vi "Translator.Translate.Text.New.vi"(6 "group":string, 8 "error in (no error)":errorcluster, 10 "text":string) -> (0 "error out":errorcluster, 2 "translated":string)   [LabVIEW 2019, in "Tools.lvlib"]
uses:
  Tools.lvlib
  TMOS config/TMOS.Config.Action.ctl
  <vilib>/Utility/config.llb/NI_LVConfig.lvlib
  Translator.File.MatchStrings (Single).vi
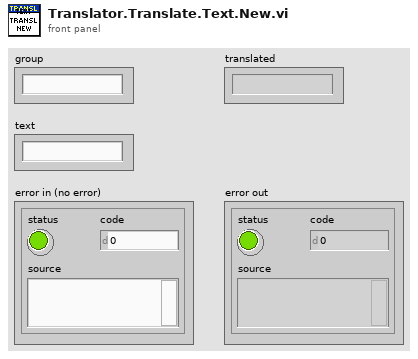
[diagram p1: front panel]
types:
  T1 = typedef "TMOS.Config.Action.ctl" = enum16{"init", "update", "get", "set"}
  T2 = typedef "NI_LVConfig.lvlib/Config Data RefNum.ctl" = refnum<k1>
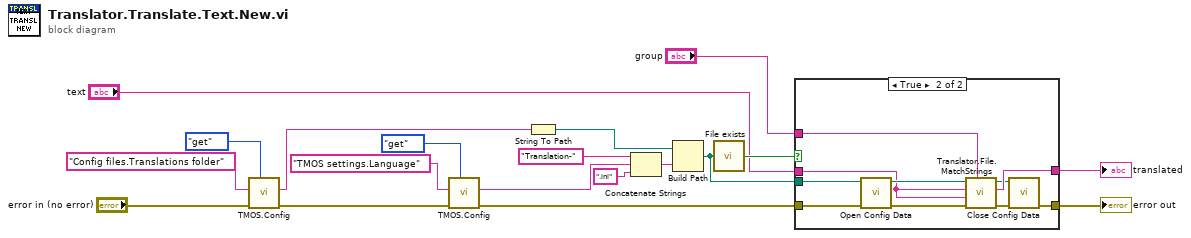
[diagram p0: block diagram]
diagram:
  n1 = call "TMOS.Config.vi"("action"=TMOS.Config.Action."get", "error in"="error in (no error)", "name"="Config files.Translations folder" ("~Language in use")) -> ("error out"=w16:errorcluster, "read value"=w13:string)  [unwired: 6 in, 1 out]
  n2 = call "TMOS.Config.vi"("action"=TMOS.Config.Action."get", "error in"=w16, "name"="TMOS settings.Language" ("~Language in use")) -> ("error out"=w4:errorcluster, "read value"=w9:string)  [unwired: 6 in, 1 out]
  n3 = String To Path(string=w13) -> (path=w8:path)
  n4 = Concatenate Strings("Translation-" ("string"), w9, ".ini" ("string")) -> (w12:string)
  n5 = Build Path(base path=w8, name or relative path=w12) -> (appended path=w5:path)
  n6 = call "File exists.vi"("file path"=w5) -> ("exists?"=w6:bool)  [unwired: 4 in]
  n7 = case shown="True" w6 {
    tunnel: w5 -> [_ w22]
    tunnel: w4 -> [w21 w31]
    tunnel: "text" -> [w20 w28]
    tunnel: [w20 w27] -> w1
    tunnel: [w21 w24] -> w2
    tunnel: "group" -> [_ w23]
    frame False {
    }
    frame True {
      n8 = call <vilib>:"Open Config Data.vi"("error in (no error)"=w31, "configuration file path"=w22) -> ("error out"=w29:errorcluster, "refnum"=w30:T2)  [unwired: 7 in, 1 out]
      n9 = call-poly "Translator.File.MatchStrings.vi"("group"=w23, "error in"=w29, "label"=w28, "default value"=w28, "refnum in"=w30) -> ("error out"=w26:errorcluster, "value out"=w27:string, "refnum out"=w25:T2)  [unwired: 3 in, 1 out]
      n10 = call <vilib>:"Close Config Data.vi"("error in (no error)"=w26, "refnum"=w25) -> ("error out"=w24:errorcluster)  [unwired: 8 in, 1 out]
    }
  }
  "error out" <- w2
  "translated" <- w1
